vi "Publish to Data Subscribers.vi"(8 "error in (no error)":errorcluster, 9 "Message Priority (Normal)":T2, 10 "Data Msg in":refnum<class "Data Msg.lvclass">, 11 "Data Subsciptions in":T1[](array[typedef])) -> (0 "error out":errorcluster, 1 "Callers found?":bool, 3 "Subsciptions out":T1[](array[typedef]))   [LabVIEW 2020, in "Publisher.lvlib" / "Publisher.lvclass"]
doc: "Get enqueuers in the hierarchy of 'Data' inside of the 'Data msg' and publish to these. All dead enqueuers are removed without throwing an error."
uses:
  Publisher.lvclass
  Messages/Data Msg/Data Msg.lvclass
  PPL/HDH.Actor Framework.Core.Actor.lvlibp/1abvi3w/vi.lib/ActorFramework/Message Enqueuer/Message Priority.ctl
  Controls/Ctl_Subscription Element.ctl
  PPL/HDH.Actor Framework.Core.Actor.lvlibp/1abvi3w/vi.lib/ActorFramework/Message Enqueuer/Message Enqueuer.lvclass
  Messages/Data Msg/Data Msg.lvclass/Data Msg.ctl
  86c92027-2f77-4d8a-9797-48f372c5338e.vi
  PPL/HDH.Data.Generic.lvlibp/Data.lvclass
  PPL/HDH.Actor Framework.Core.Utility.lvlibp
  C:/Current projects/WS/PPL/HDH.Actor Framework.Core.Actor.lvlibp/1abvi3w/vi.lib/ActorFramework/Message/Message.lvclass
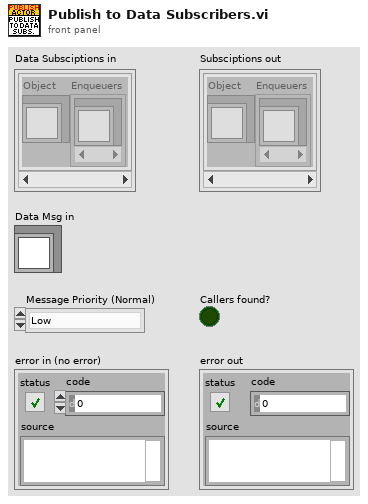
[diagram p1: front panel]
types:
  T1 = typedef "Publisher.lvlib/Publisher.lvclass/Ctl_Subscription Element.ctl" = cluster{"Object":refnum<class>, "Enqueuers":refnum<class "Message Enqueuer.lvclass">[]}
  T2 = typedef "HDH.Actor Framework.Core.Actor.lvlibp/Message Enqueuer.lvclass/Message Priority.ctl" = enum16{"Low", "Normal", "High"}
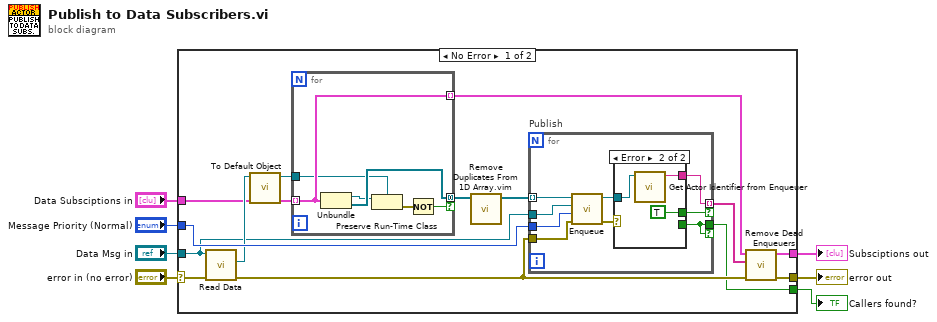
[diagram p0: block diagram]
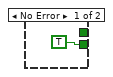
[diagram p2: hidden frame]
diagram:
  n1 = case shown="No Error" "error in (no error)" {
    selector: "error in (no error)" -> [w13 w42]
    tunnel: [w21 w42] -> w7
    tunnel: "Message Priority (Normal)" -> [w20 _]
    tunnel: "Data Msg in" -> [w11 _]
    tunnel: "Data Subsciptions in" -> [w10 w41]
    tunnel: [w15 w41] -> w3
    tunnel: [w8 _] -> w1
    frame No Error {
      n2 = call "Read Data.vi"("error in (no error)"=w13, "Data Msg in"=w11) -> ("error out"=w12:errorcluster, "Data"=w14:refnum<class "Data.lvclass">)  [unwired: 7 in, 1 out]
      n3 = call "To Default Object.vi"("Object in"=w14) -> ("Default out"=w19:refnum<class "Data.lvclass">)  [unwired: 10 in]
      n4 = for {
        tunnel: w19 -> [w22]
        tunnel: w10 -> [w24] mode=indexing
        tunnel: [w26] -> w18 mode=concatenating if=w25
        tunnel: [w24] -> w9 mode=indexing
        n5 = Unbundle(w24) -> ("Object"=w23:refnum<class>, "Enqueuers"=w26:refnum<class "Message Enqueuer.lvclass">[])
        n6 = Preserve Run-Time Class(object in=w23, 2:w22) -> (error out=w27:errorcluster)  [unwired: 1 in, 1 out]
        n7 = Not(x=w27) -> (.not. x?=w25:bool)
      }
      n8 = call "Remove Duplicates From 1D Array.vim"("array"=w18) -> ("array with duplicates removed"=w17:refnum<class "Message Enqueuer.lvclass">[])  [unwired: 10 in]
      n9 = for "Publish" {
        tunnel: w17 -> [w36] mode=indexing
        tunnel: w20 -> [w35]
        tunnel: w11 -> [w34]
        tunnel: [w31] -> w16 mode=indexing if=w30
        tunnel: w12 -> [w29]
        tunnel: [w28] -> w8 if=w28
        n10 = call "Enqueue.vi"("error in (no error)"=w29, "Message Priority (Normal)"=w35, "Message"=w34, "Message Enqueuer in"=w36) -> ("error out"=w33:errorcluster, "Message Enqueuer out"=w32:refnum<class "Message Enqueuer.lvclass">)  [unwired: 6 in]
        n11 = case shown="Error" w33 {
          tunnel: w32 -> [_ w40]
          tunnel: [_ w39] -> w31
          tunnel: [_ TRUE] -> w30
          tunnel: [TRUE _] -> w28
          frame No Error {
          }
          frame Error {
            n12 = call "Get Actor Identifier from Enqueuer.vi"("Message Enqueuer in"=w40) -> ("Actor ID string out"=w39:string)  [unwired: 9 in, 1 out]
          }
        }
      }
      n13 = call "Remove Dead Enqueuers.vi"("error in (no error)"=w12, "Enqueuers to remove"=w16, "Subsciptions in"=w9) -> ("error out"=w21:errorcluster, "Subsciptions out"=w15:T1[])  [unwired: 7 in]
    }
    frame Error {
    }
  }
  "error out" <- w7
  "Subsciptions out" <- w3
  "Callers found?" <- w1
